vi "Initialize.vi"(8 "error in (no error)":errorcluster, 11 "View Template in":refnum<class "[MV] Key Generator.lvclass">) -> (0 "error out":errorcluster, 3 "View Template out":refnum<class "[MV] Key Generator.lvclass">)   [LabVIEW 2020, in "[MV] Key Generator.lvlib" / "[MV] Key Generator.lvclass"]
uses:
  [MV] Key Generator.lvclass
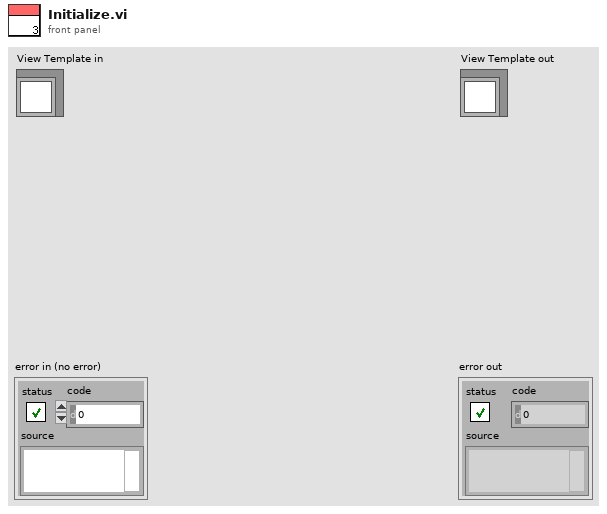
[diagram p1: front panel]
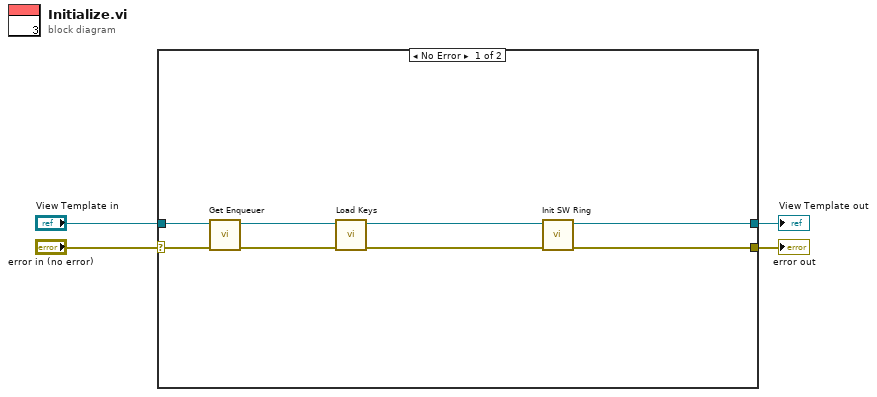
[diagram p0: block diagram]
diagram:
  n1 = case shown="No Error" "error in (no error)" {
    selector: "error in (no error)" -> [w11 w14]
    tunnel: [w7 w14] -> w3
    tunnel: [w5 w13] -> w1
    tunnel: "View Template in" -> [w12 w13]
    frame No Error {
      n2 = call "Get Enqueuer.vi"("error in (no error)"=w11, "View Template in"=w12) -> ("error out"=w10:errorcluster, "View Template out"=w8:refnum<class "[MV] Key Generator.lvclass">)  [unwired: 8 in]
      n3 = call "Load Keys.vi"("error in (no error)"=w10, "[MV] Key Generator in"=w8) -> ("error out"=w9:errorcluster, "[MV] Key Generator out"=w6:refnum<class "[MV] Key Generator.lvclass">)  [unwired: 8 in]
      n4 = call "Init SW Ring.vi"("error in (no error)"=w9, "[MV] Key Generator in"=w6) -> ("error out"=w7:errorcluster, "[MV] Key Generator out"=w5:refnum<class "[MV] Key Generator.lvclass">)  [unwired: 8 in]
    }
    frame Error {
    }
  }
  "error out" <- w3
  "View Template out" <- w1
